vi "VarOperator.vi"(6 "Data Type":T1, 7 "ro/w/r":T2=enum."Read Only", 8 "error in":errorcluster, 9 "Data":i64, 10 "PDO Name":string, 11 "Motor Base in":refnum<class "Motor Base.lvclass">) -> (0 "error out":errorcluster, 2 "Data":i64, 3 "Motor Base out":refnum<class "Motor Base.lvclass">, 4 "Time Stamp":timestamp, 5 "shared variable refnum out":refnum<k21>)   [LabVIEW 2016, in "Motor Base.lvlib" / "Motor Base.lvclass"]
uses:
  Motor Base.lvclass
  AccessType.ctl
  Data Type.ctl
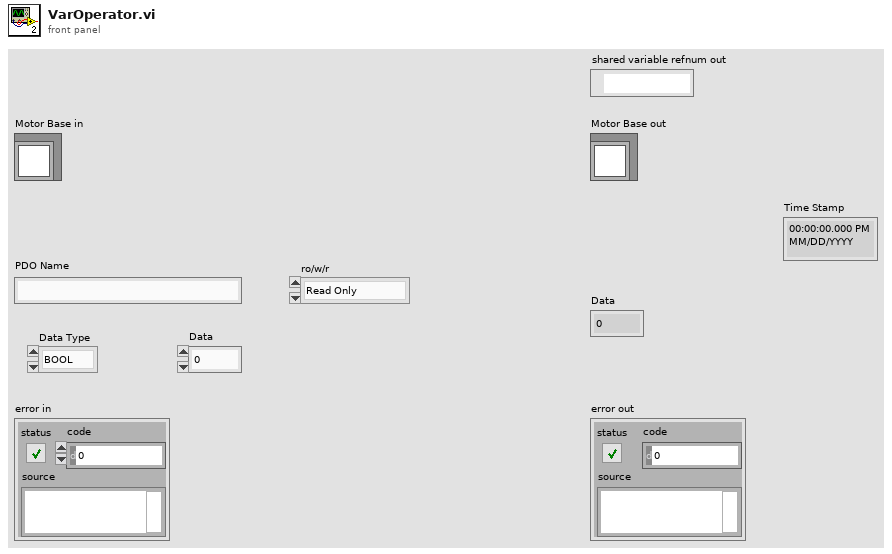
[diagram p1: front panel]
types:
  T1 = typedef "Motor Base.lvlib/Motor Base.lvclass/Data Type.ctl" = enum16{"BOOL", "I16", "I32", "I8", "OS", "U16", "U32", "U8", "VS"}
  T2 = typedef "Motor Base.lvlib/Motor Base.lvclass/AccessType.ctl" = enum16{"Write", "Read", "Read Only"}
  T3 = cluster{"Pre_String":string, "Target Name":string, "Master Name":string, "Device Name":string}
  T4 = cluster{"Pre_String":string, "Target Name":string, "Master Name":string, "Device Name":string, "PDO Mapping R":string, "PDO Mapping T":string}
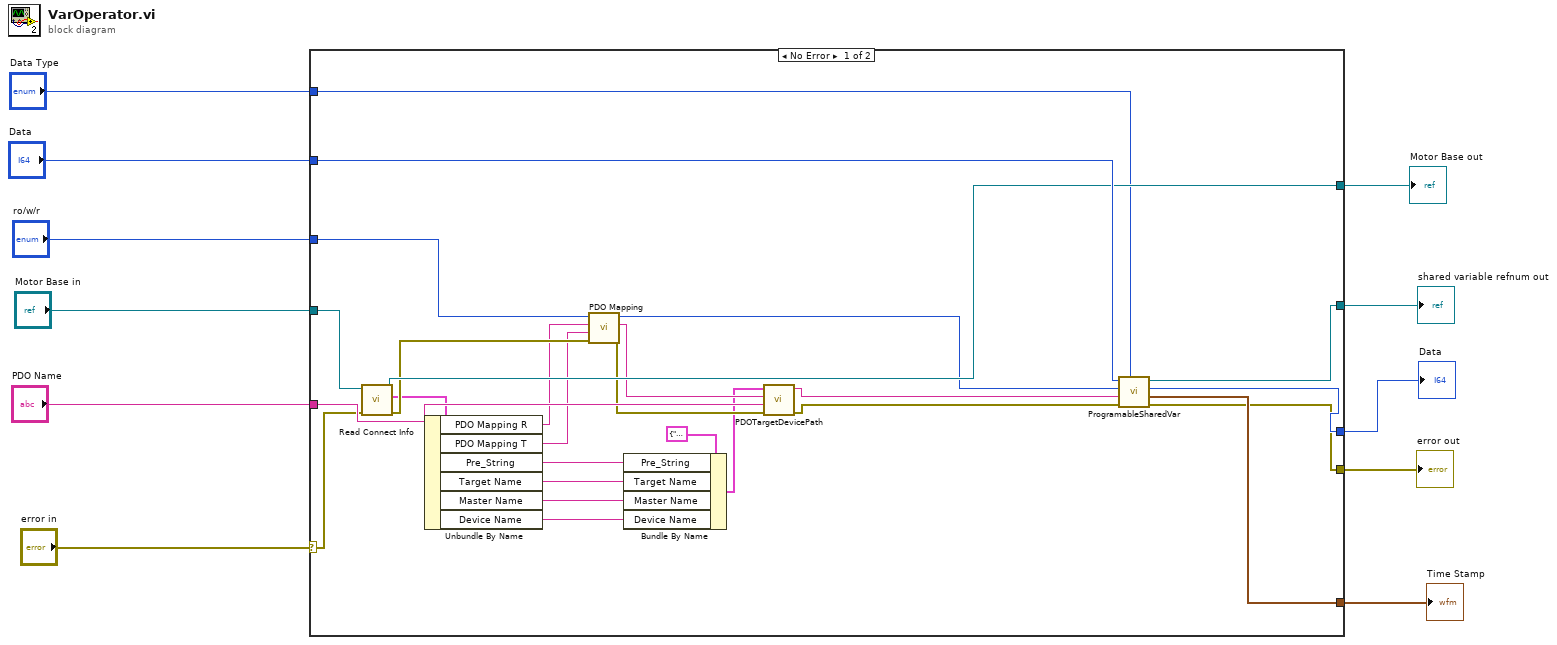
[diagram p0: block diagram]
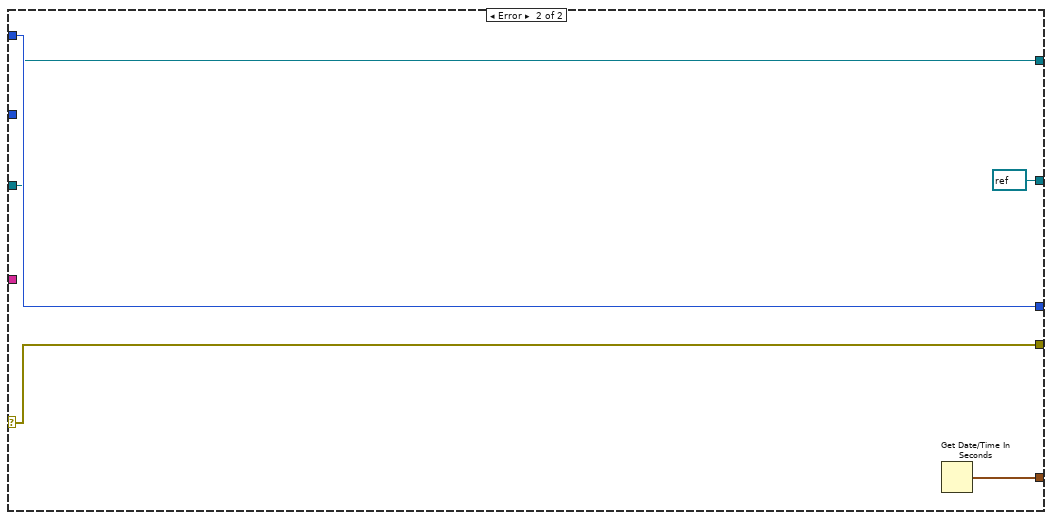
[diagram p2: hidden frame]
diagram:
  n1 = case shown="No Error" "error in" {
    selector: "error in" -> [w28 w42]
    tunnel: "PDO Name" -> [w37 _]
    tunnel: "ro/w/r" -> [w25 _]
    tunnel: [w35 w40] -> w9
    tunnel: [w33 w41] -> w8
    tunnel: [w32 w42] -> w7
    tunnel: [w31 refnum<k21> refnum ("PDO Path")] -> w2
    tunnel: "Data" -> [w30 w40]
    tunnel: "Motor Base in" -> [w29 w39]
    tunnel: [w27 w39] -> w3
    tunnel: "Data Type" -> [w12 _]
    frame No Error {
      n2 = call-dynamic "Read Connect Info.vi"("error in (no error)"=w28, "Motor Base in"=w29) -> ("error out"=w23:errorcluster, "Connect Info"=w21:T4, "Motor Base out"=w27:refnum<class "Motor Base.lvclass">)  [unwired: 7 in]
      n3 = Unbundle By Name(w21) -> ("PDO Mapping R"=w14:string, "PDO Mapping T"=w13:string, "Pre_String"=w18:string, "Target Name"=w17:string, "Master Name"=w16:string, "Device Name"=w15:string)
      n4 = call "PDO Mapping.vi"("error in"=w23, "PDO Mapping T"=w13, "PDO Mapping R"=w14, "ro/r/w"=w25) -> ("error out"=w22:errorcluster, "PDO Mapping"=w26:string, "ro/r/w"=w24:T2)  [unwired: 5 in]
      n5 = Bundle By Name(cluster=T3 {"Pre_String"="ni.var.io", "Target Name"="RT PXI Target", "Master Name"="EtherCAT Master", "Device Name"="Device"} ("PDOTargetDevicePath"), "Pre_String"=w18, "Target Name"=w17, "Master Name"=w16, "Device Name"=w15) -> (w19:T3)
      n6 = call "PDOTargetDevicePath.vi"("error in (no error)"=w22, "PDO Name"=w37, "PDO Mapping"=w26, "PDOTargetDevicePath"=w19) -> ("error out"=w34:errorcluster, "String"=w36:string)  [unwired: 6 in]
      n7 = call "ProgramableSharedVar.vi"("Data Type"=w12, "error in (no error)"=w34, "String"=w36, "ro/r/w"=w24, "Data in"=w30) -> ("error out"=w32:errorcluster, "TimeStamp"=w33:timestamp, "Data out"=w35:i64, "PDO Path"=w31:refnum<k21>)  [unwired: 3 in]
    }
    frame Error {
      n8 = Get Date/Time In Seconds() -> (seconds since 1Jan1904=w41:timestamp)
    }
  }
  "error out" <- w7
  "Data" <- w9
  "Time Stamp" <- w8
  "Motor Base out" <- w3
  "shared variable refnum out" <- w2
